vi "Load_Limits.vi"(10 "error in (no error)":errorcluster) -> (2 "error out":errorcluster, 5 "limits ok?":bool, 9 "all rows":string[][](array[string]), 11 "Limits":T1)   [LabVIEW 2026]
uses:
  <vilib>/Utility/file.llb/Read Delimited Spreadsheet (string).vi
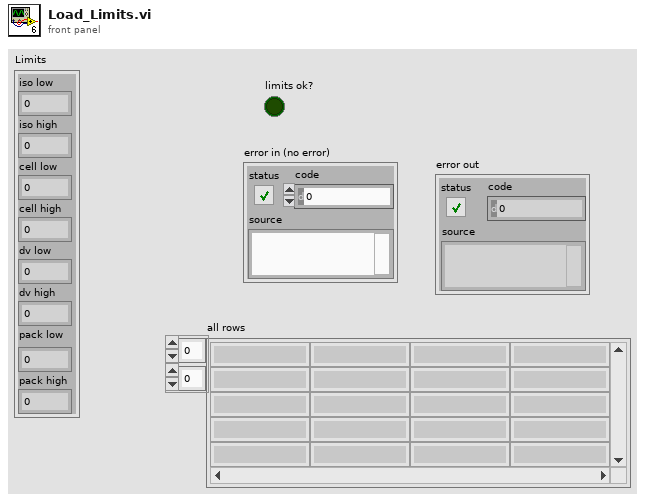
[diagram p1: front panel]
types:
  T1 = cluster{"iso low":dbl, "iso high":dbl, "cell low":dbl, "cell high":dbl, "dv low":dbl, "dv high":dbl, "pack low":dbl, "pack high":dbl}
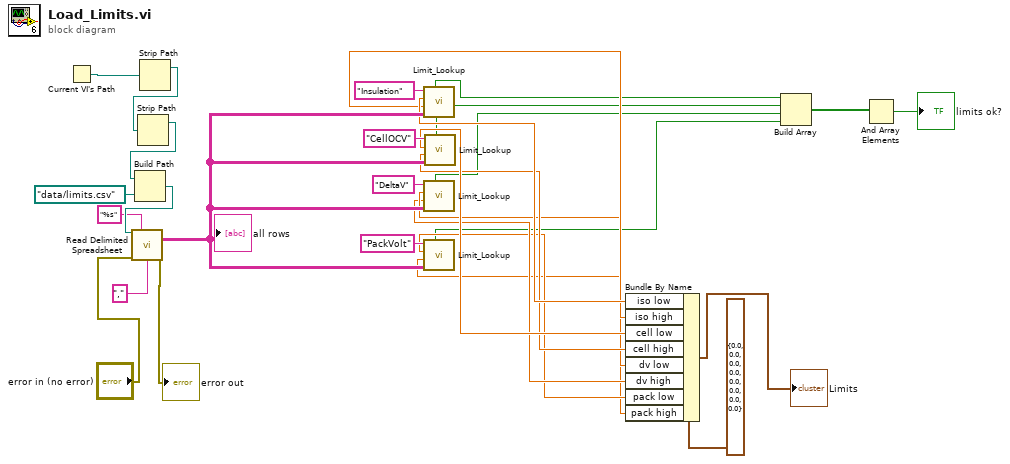
[diagram p0: block diagram]
diagram:
  n1 = Current VI's Path() -> (path=w29:path)
  n2 = Strip Path(path=w29) -> (stripped path=w30:path)  [unwired: 1 out]
  n3 = Strip Path(path=w30) -> (stripped path=w28:path)  [unwired: 1 out]
  n4 = Build Path(base path=w28, name or relative path=path "data/limits.csv") -> (appended path=w26:path)
  n5 = call-poly <vilib>:"Read Delimited Spreadsheet.vi"("file path (dialog if empty)"=w26, "format (%s)"="%s", "error in (no error)"="error in (no error)", "delimiter (\\t)"="," ("delimiter (\\t)")) -> ("all rows"=w23:string[][], "error out"=→"error out":errorcluster)  [unwired: 6 in, 4 out]
  "all rows" <- w23
  n6 = call "Limit_Lookup.vi"("all rows"=w23, "step name"="Insulation") -> ("found?"=w9:bool, "high"=w16:dbl, "low"=w17:dbl)  [unwired: 7 in]
  n7 = call "Limit_Lookup.vi"("all rows"=w23, "step name"="DeltaV") -> ("found?"=w7:bool, "high"=w12:dbl, "low"=w13:dbl)  [unwired: 7 in]
  n8 = call "Limit_Lookup.vi"("all rows"=w23, "step name"="PackVolt") -> ("found?"=w6:bool, "high"=w10:dbl, "low"=w11:dbl)  [unwired: 7 in]
  n9 = call "Limit_Lookup.vi"("all rows"=w23, "step name"="CellOCV") -> ("found?"=w8:bool, "high"=w14:dbl, "low"=w15:dbl)  [unwired: 7 in]
  n10 = Bundle By Name(cluster=T1 {"iso low"=0.0, "iso high"=0.0, "cell low"=0.0, "cell high"=0.0, "dv low"=0.0, "dv high"=0.0, "pack low"=0.0, "pack high"=0.0} ("Limits 2"), "iso low"=w17, "iso high"=w16, "cell low"=w15, "cell high"=w14, "dv low"=w13, "dv high"=w12, "pack low"=w11, "pack high"=w10) -> (→"Limits":T1)
  n11 = Build Array(w9, w8, w7, w6) -> (w5:bool[])
  n12 = And Array Elements(Boolean array=w5) -> (logical AND=→"limits ok?":bool)
